vi "电机定位1.1.vi"(0 "VISA I":refnum<visa-resource-name>, 1 "等待时间(ms)":u32=40, 2 "细分设置":dbl=8.0, 3 "电机急停":bool, 4 "X":dbl, 5 "精度":dbl=0.001, 6 "pulDDR2Length":u32, 8 "hDevice":i32, 10 "M-length":dbl, 12 "N-length":dbl) -> (13 "hDevice out":i32, 14 "VISA O":refnum<visa-resource-name>, 18 "X":dbl, 19 "Y":dbl)   [LabVIEW 2016]
uses:
  <vilib>/Analysis/2dsp.llb/Real FFT.vi
  <vilib>/Analysis/4window.llb/Gaussian Window (DBL).vi
  <vilib>/Utility/file.llb/Write Delimited Spreadsheet (DBL).vi
  <vilib>/Utility/file.llb/Read Delimited Spreadsheet (DBL).vi
  <vilib>/Analysis/NI_AALBase.lvlib
  <vilib>/Analysis/NI_AALPro.lvlib
panel:
  out "有效值":dbl
  out "空扫底噪":cdb[](array[numeric])
  out "采集卡底噪":cdb[](array[numeric])
  in  "保存信号":bool
  out "幅频谱":dbl[](graph)
  out "时域谱":dbl[](graph)
  in  "查询信号":bool
  in  "Y":dbl
  in  "确定":bool
  in  "ESC":bool
  # "时域谱"
  # "频域谱"
  # "目标位置"
  # "实时位置"
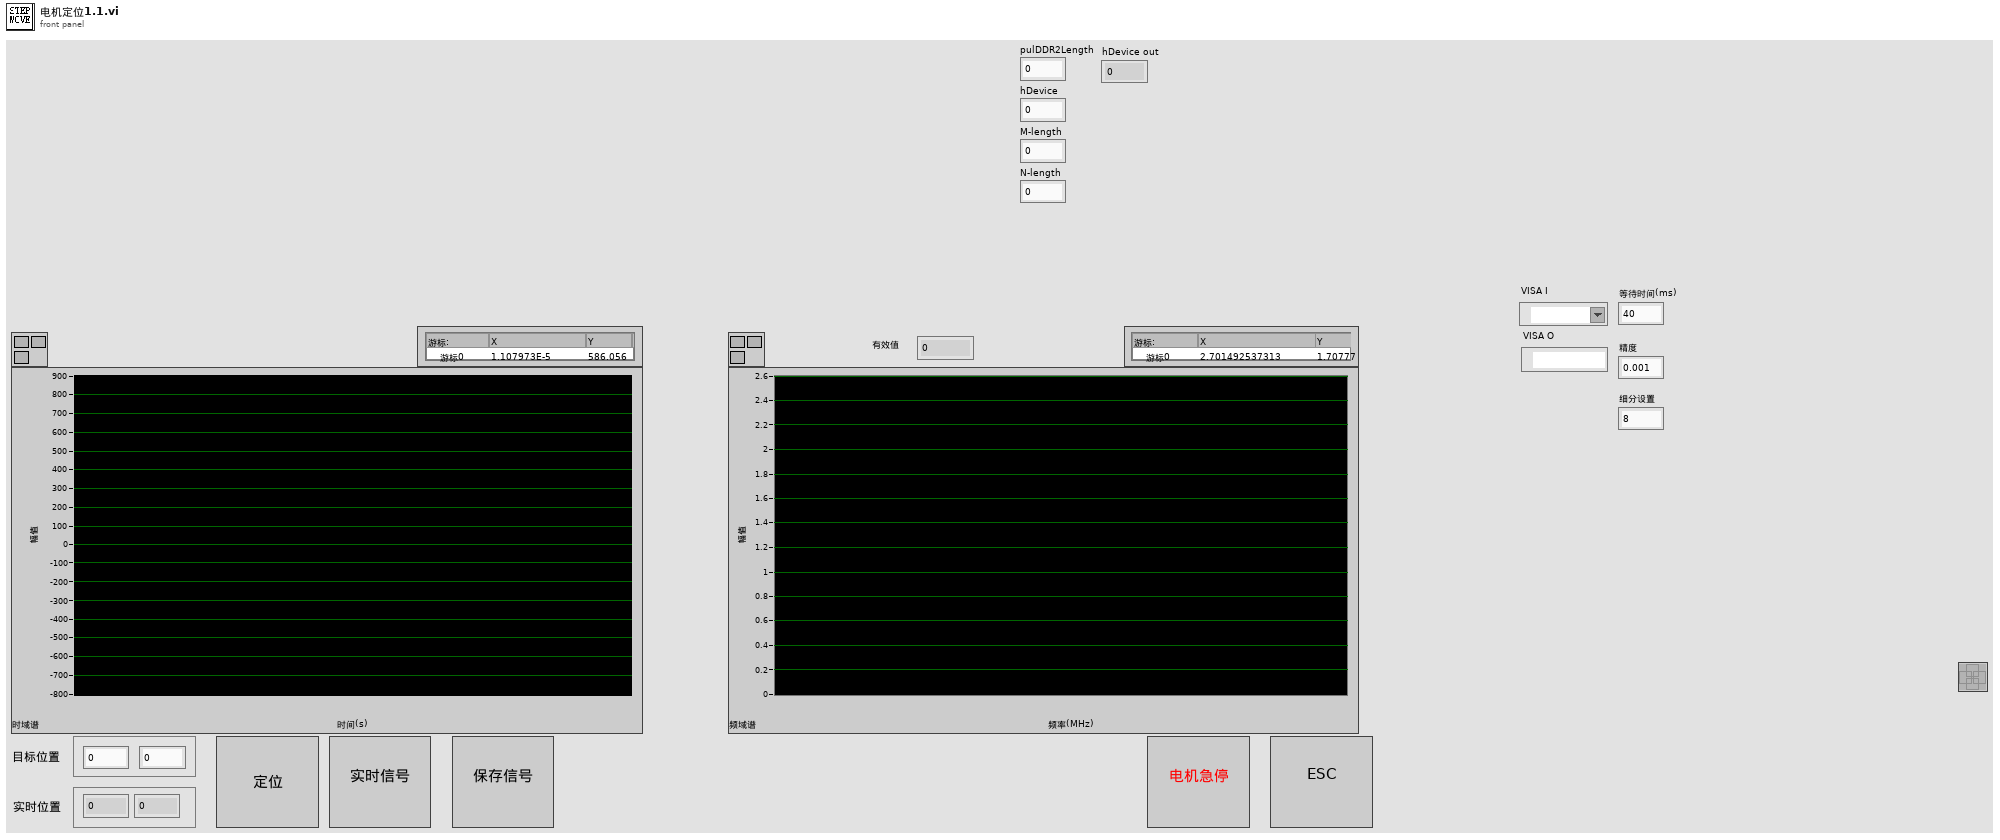
[diagram p1: front panel]
types:
  T1 = enum16{"open", "replace", "create", "open or create", "replace or create", "replace or create with confirmation"}
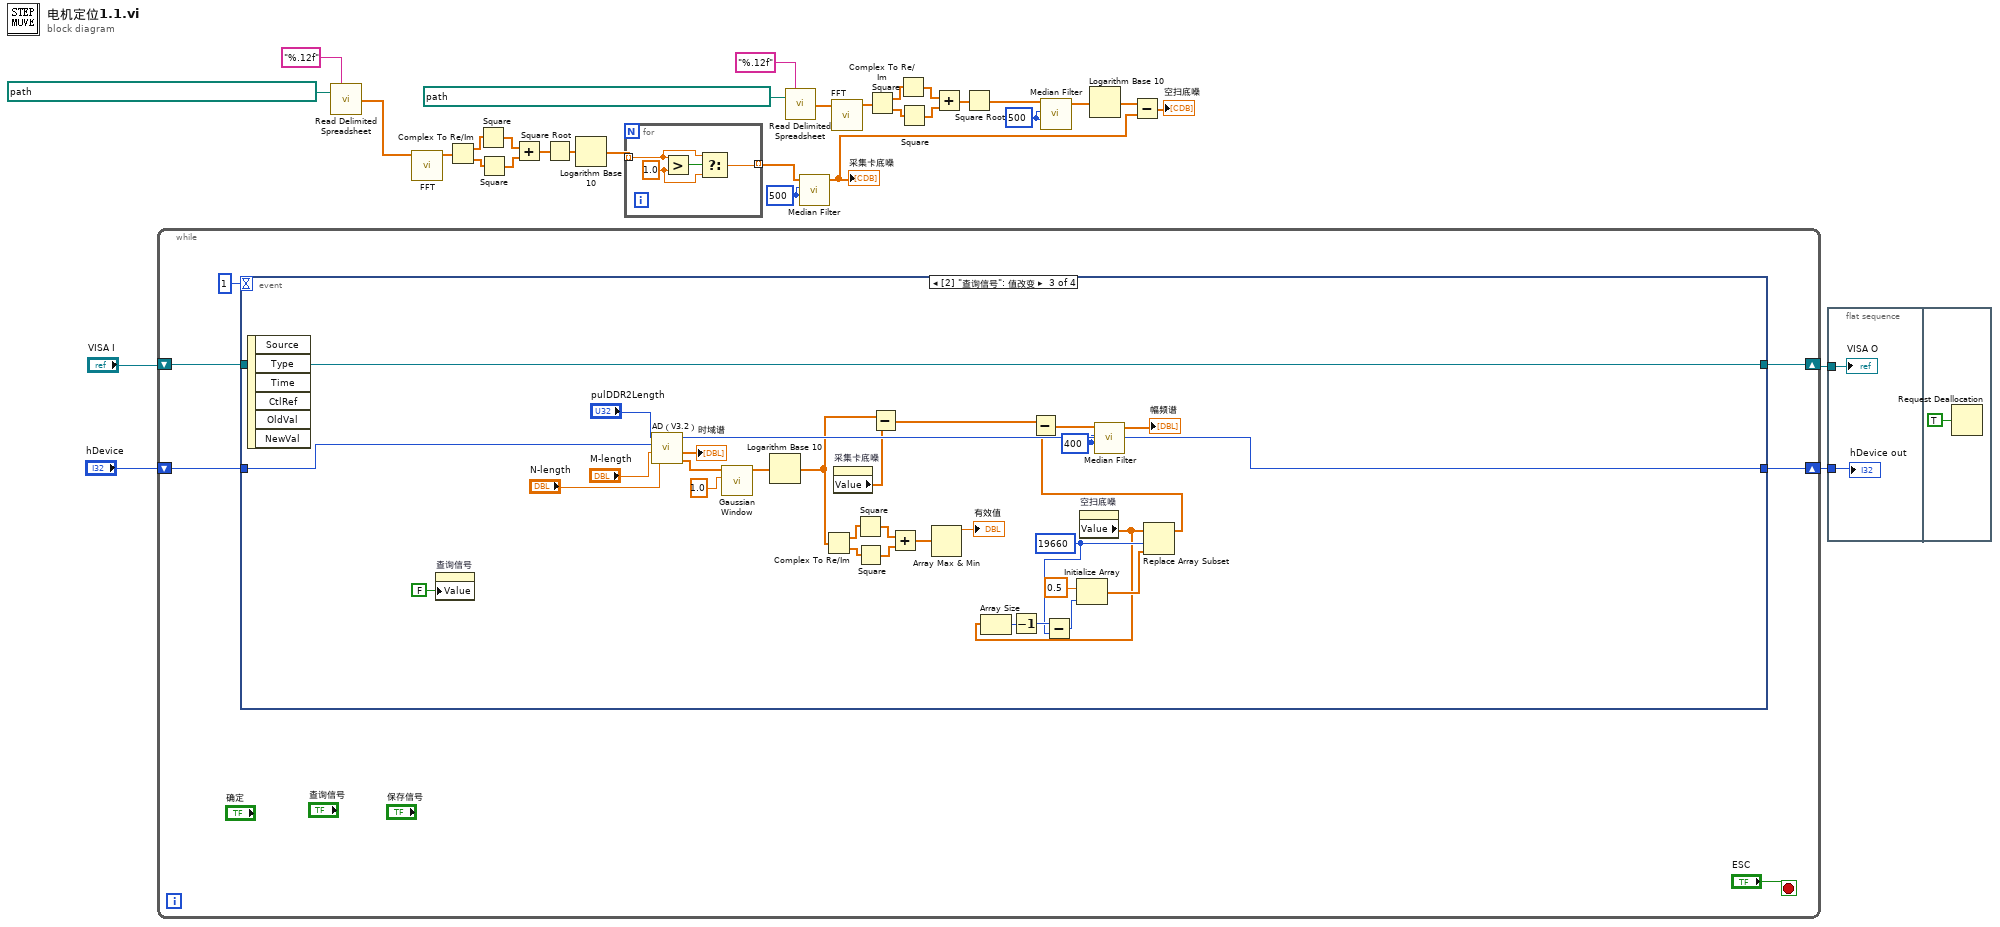
[diagram p0: block diagram]
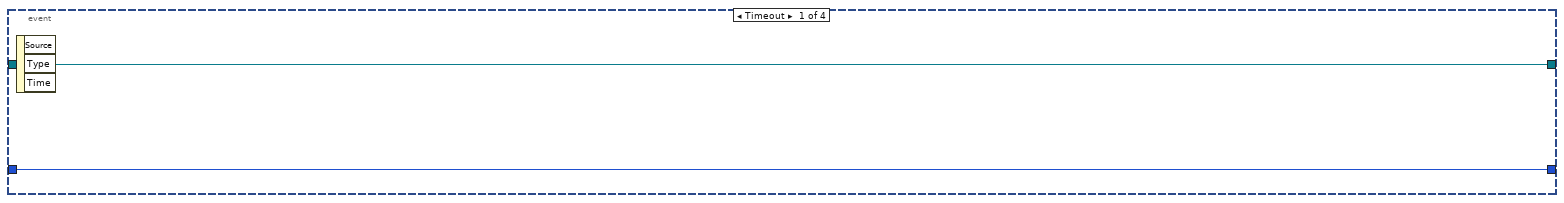
[diagram p2: hidden frame]
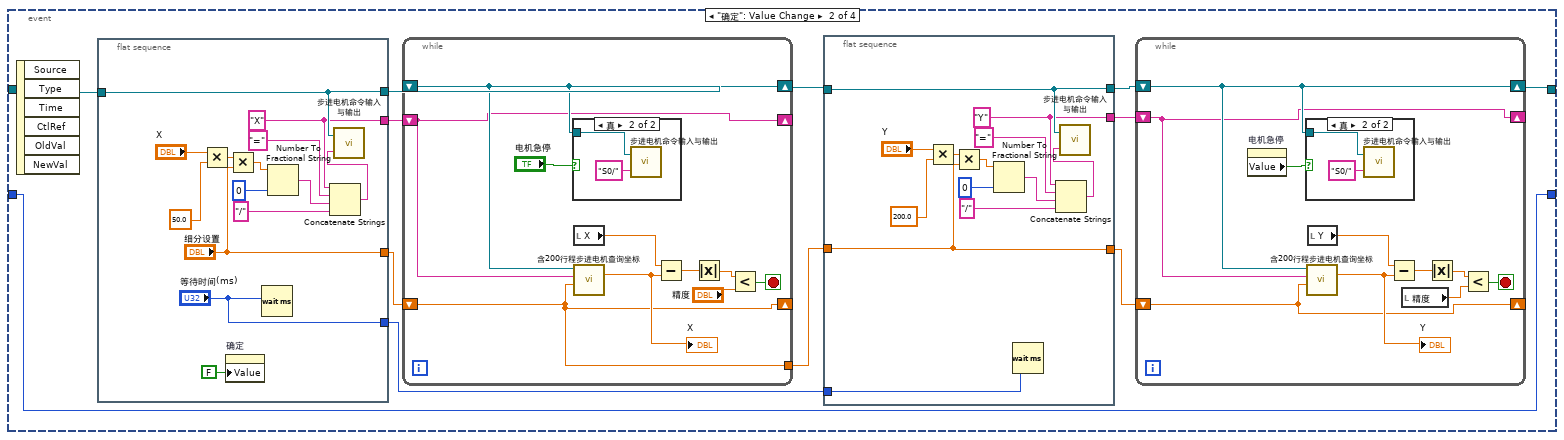
[diagram p3: hidden frame]
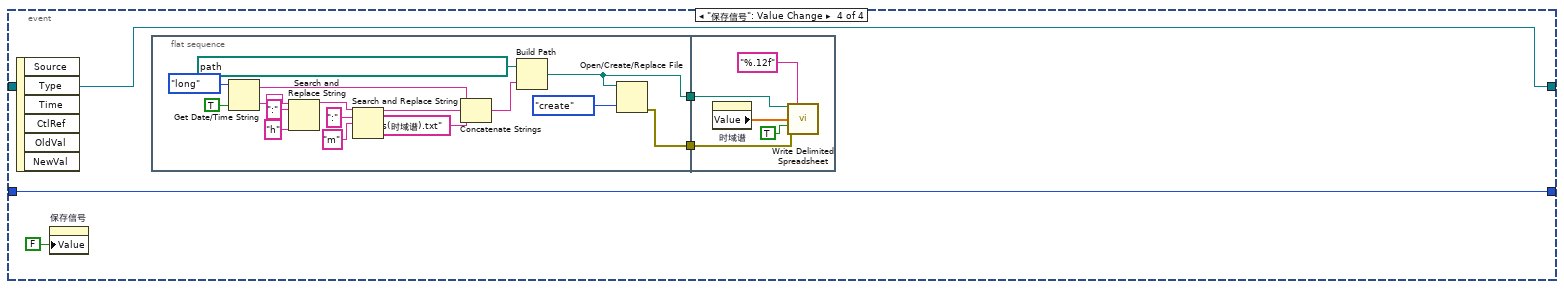
[diagram p6: hidden frame]
diagram:
  w8 = 500 ("left rank")
  w26 = 500 ("left rank")
  n1 = while {
    shift-right: [w37] -> w32
    shift-left: "VISA I" -> [w38]
    shift-right: [w34] -> w29
    shift-left: "hDevice" -> [w35]
    stop <- "ESC" stop-if-true
    n2 = event shown="[2] \"查询信号\": 值改变" {
      selector: _ -> [_ _ _ _]
      dyn-events: _ -> [_ _ _ _]
      timeout: 1 -> [_ _ _ _]
      tunnel: w38 -> [w40 w52 w134 w138]
      tunnel: [w40 w51 w134 w138] -> w37
      tunnel: w35 -> [w39 w41 w130 w137]
      tunnel: [w39 w41 w129 w137] -> w34
      event Timeout {
        n3 = event-data() -> ()  [unwired: 1 in, 3 out]
      }
      event "确定": Value Change {
        n4 = event-data() -> ()  [unwired: 1 in, 6 out]
        n5 = flat-sequence {
          tunnel: w52 -> [w95]
          tunnel: [w95] -> w50
          tunnel: ["细分设置"] -> w49
          tunnel: [w92] -> w48
          tunnel: ["等待时间(ms)"] -> w43
          frame #0 {
            w92 = "X"
            n6 = Multiply(x="X", y=50.0 ("x")) -> (x*y=w98:dbl)
            n7 = property on="确定" class="Bool (严格)"("Value"=FALSE ("确定")) -> ()  [unwired: 2 in, 2 out]
            n8 = Multiply(x=w98, y="细分设置") -> (x*y=w103:dbl)
            n9 = Wait (ms)(milliseconds to wait="等待时间(ms)") -> ()  [unwired: 1 out]
            n10 = Number To Fractional String(number=w103, precision (6)=i16 0 ("精度(6)")) -> (F-format string=w101:string)  [unwired: 2 out]
            n11 = Concatenate Strings(w92, "=" ("字符串"), w101, "/" ("字符串")) -> (w97:string)
            n12 = call "步进电机命令输入与输出.vi"("输入字符串"=w97, "串口通信端口"=w95) -> ()  [unwired: 1 out]
          }
        }
        n13 = while {
          tunnel: [w78] -> w42
          shift-right: [w84] -> w44
          shift-left: w50 -> [w84]
          shift-right: [w79] -> _
          shift-left: w48 -> [w79]
          shift-right: [w78] -> _
          shift-left: w49 -> [w78]
          stop <- w87 stop-if-true
          n14 = case shown="真" "电机急停" {
            tunnel: w84 -> [_ w88]
            frame False {
            }
            frame True {
              n15 = call "步进电机命令输入与输出.vi"("输入字符串"="S0/", "串口通信端口"=w88) -> ()  [unwired: 1 out]
            }
          }
          n16 = local read "X"() -> (w82:dbl)
          n17 = call "含200行程步进电机查询坐标.vi"("细分设置"=w78, "查询坐标轴"=w79, "串口通信端口"=w84) -> ("坐标(mm)"=w81:dbl)  [unwired: 8 in]
          "X" <- w81
          n18 = Subtract(x=w82, y=w81) -> (x-y=w86:dbl)
          n19 = Absolute Value(x=w86) -> (abs(x)=w85:dbl)
          n20 = Less?(x=w85, y="精度") -> (x < y?=w87:bool)
        }
        n21 = flat-sequence {
          tunnel: w44 -> [w69]
          tunnel: [w69] -> w47
          tunnel: [w65] -> w46
          tunnel: [w67] -> w45
          tunnel: w43 -> [w66]
          tunnel: w42 -> [w65]
          frame #0 {
            w67 = "Y"
            n22 = Multiply(x="Y", y=200.0 ("x")) -> (x*y=w72:dbl)
            n23 = Multiply(x=w72, y=w65) -> (x*y=w77:dbl)
            n24 = Number To Fractional String(number=w77, precision (6)=i16 0 ("精度(6)")) -> (F-format string=w75:string)  [unwired: 2 out]
            n25 = Wait (ms)(milliseconds to wait=w66) -> ()  [unwired: 1 out]
            n26 = Concatenate Strings(w67, "=" ("字符串"), w75, "/" ("字符串")) -> (w71:string)
            n27 = call "步进电机命令输入与输出.vi"("输入字符串"=w71, "串口通信端口"=w69) -> ()  [unwired: 1 out]
          }
        }
        n28 = while {
          shift-right: [w59] -> w51
          shift-left: w47 -> [w59]
          shift-right: [w54] -> _
          shift-left: w45 -> [w54]
          shift-right: [w53] -> _
          shift-left: w46 -> [w53]
          stop <- w62 stop-if-true
          n29 = property on="电机急停" class="Bool (严格)"() -> ("Value"=w55:bool)  [unwired: 2 in, 2 out]
          n30 = case shown="真" w55 {
            tunnel: w59 -> [_ w63]
            frame False {
            }
            frame True {
              n31 = call "步进电机命令输入与输出.vi"("输入字符串"="S0/", "串口通信端口"=w63) -> ()  [unwired: 1 out]
            }
          }
          n32 = call "含200行程步进电机查询坐标.vi"("细分设置"=w53, "查询坐标轴"=w54, "串口通信端口"=w59) -> ("坐标(mm)"=w57:dbl)  [unwired: 8 in]
          "Y" <- w57
          n33 = local read "Y"() -> (w58:dbl)
          n34 = Subtract(x=w58, y=w57) -> (x-y=w61:dbl)
          n35 = local read "精度"() -> (w56:dbl)
          n36 = Absolute Value(x=w61) -> (abs(x)=w60:dbl)
          n37 = Less?(x=w60, y=w56) -> (x < y?=w62:bool)
        }
      }
      event "查询信号": Value Change {
        w109 = 19660 ("索引")
        w127 = 400 ("left rank")
        n38 = event-data() -> ()  [unwired: 1 in, 6 out]
        n39 = property on="查询信号" class="Bool (严格)"("Value"=FALSE ("查询信号")) -> ()  [unwired: 2 in, 2 out]
        n40 = call "AD（V3.2）.vi"("N-length"="N-length", "M-length"="M-length", "hDevice"=w130, "pulDDR2Length"="pulDDR2Length") -> ("幅频谱"=w114:dbl[], "时域谱"=→"时域谱":dbl[], "hDevice out"=w129:i32)  [unwired: 5 in]
        n41 = call-poly <vilib>:"Gaussian Window.vi"("standard deviation"=1.0, "X"=w114) -> ("Windowed X"=w113:dbl[])  [unwired: 8 in, 1 out]
        n42 = Logarithm Base 10(1:w113) -> (0:w117:dbl[])
        n43 = Complex To Re/Im(x + iy=w117) -> (x=w122:dbl[], y=w123:dbl[])
        n44 = property on="采集卡底噪" class="Arr (严格)"() -> ("Value"=w116:cdb[])  [unwired: 2 in, 2 out]
        n45 = Square(x=w122) -> (x^2=w124:dbl[])
        n46 = Square(x=w123) -> (x^2=w125:dbl[])
        n47 = Subtract(x=w117, y=w116) -> (x-y=w119:cdb[])
        n48 = Add(x=w124, y=w125) -> (x+y=w121:dbl[])
        n49 = Array Max & Min(array=w121) -> (max value=→"有效值":dbl)  [unwired: 3 out]
        n50 = property on="空扫底噪" class="Arr (严格)"() -> ("Value"=w106:cdb[])  [unwired: 2 in, 2 out]
        n51 = Array Size(array=w106) -> (size(s)=w111:i32)
        n52 = Decrement(x=w111) -> (x-1=w110:i32)
        n53 = Subtract(x=w110, y=w109) -> (x-y=w108:i32)
        n54 = Initialize Array(0.5 ("元素"), w108) -> (w107:dbl[])
        n55 = Replace Array Subset(array=w106, new element=w107, index=w109) -> (w105:cdb[])
        n56 = Subtract(x=w119, y=w105) -> (x-y=w115:cdb[])
        n57 = call <vilib>:"Median Filter.vi"("right rank"=w127, "left rank"=w127, "X"=w115) -> ("Filtered X"=→"幅频谱":dbl[])  [unwired: 7 in, 1 out]
      }
      event "保存信号": Value Change {
        n58 = event-data() -> ()  [unwired: 1 in, 6 out]
        n59 = property on="保存信号" class="Bool (严格)"("Value"=FALSE ("保存信号")) -> ()  [unwired: 2 in, 2 out]
        n60 = flat-sequence {
          tunnel: [w153] -> w136
          tunnel: [w152] -> w135
          tunnel: w136 -> [w157]
          tunnel: w135 -> [w156]
          frame #0 {
            n61 = Get Date/Time String(date format (0)=enum16{"short", "long", "abbreviated"}."long" ("日期格式(0)"), want seconds? (F)=TRUE ("需要秒？(F)")) -> (date string=w144:string, time string=w145:string)  [unwired: 1 in]
            n62 = Search and Replace String(input string=w145, search string=":" ("搜索字符串"), replace string="h" ("替换字符串(\"\")")) -> (result string=w150:string)  [unwired: 5 in, 3 out]
            n63 = Search and Replace String(input string=w150, search string=":" ("搜索字符串"), replace string="m" ("替换字符串(\"\")")) -> (result string=w143:string)  [unwired: 5 in, 3 out]
            n64 = Concatenate Strings(w144, w143, "s(时域谱).txt" ("字符串")) -> (w142:string)
            n65 = Build Path(base path=path "C:/Users/H301/Desktop/art采集实验数据/单点时域谱" ("基路径"), name or relative path=w142) -> (appended path=w153:path)
            n66 = Open/Create/Replace File(file path (use dialog)=w153, operation (0:open)=T1."create" ("操作(0:open)")) -> (error out=w152:errorcluster)  [unwired: 4 in, 2 out]
          }
          frame #1 {
            n67 = property on="时域谱" class="WFGraph (严格)"() -> ("Value"=w158:dbl[])  [unwired: 2 in, 2 out]
            n68 = call-poly <vilib>:"Write Delimited Spreadsheet.vi"("file path (dialog if empty)"=w157, "format (%.3f)"="%.12f", "1D data"=w158, "append to file? (new file:F)"=TRUE, "error in (no error)"=w156) -> ()  [unwired: 9 in, 2 out]
          }
        }
      }
    }
  }
  n69 = call-poly <vilib>:"Read Delimited Spreadsheet.vi"("file path (dialog if empty)"=path "C:/Users/H301/Desktop/art采集实验数据/采集卡均值底噪.txt", "format (%.3f)"="%.12f") -> ("first row"=w9:dbl[])  [unwired: 8 in, 5 out]
  n70 = call-poly <vilib>:"FFT.vi"("X"=w9) -> ("FFT {X}"=w12:cdb[])  [unwired: 9 in, 1 out]
  n71 = Complex To Re/Im(x + iy=w12) -> (x=w10:dbl[], y=w11:dbl[])
  n72 = Square(x=w10) -> (x^2=w13:dbl[])
  n73 = Square(x=w11) -> (x^2=w14:dbl[])
  n74 = Add(x=w13, y=w14) -> (x+y=w15:dbl[])
  n75 = Square Root(x=w15) -> (sqrt(x)=w6:dbl[])
  n76 = Logarithm Base 10(1:w6) -> (0:w5:dbl[])
  n77 = for {
    tunnel: w5 -> [w162] mode=indexing
    tunnel: [w161] -> w7 mode=indexing
    w163 = 1.0 ("y")
    n78 = Greater?(x=w162, y=w163) -> (0:w164:bool)
    n79 = Select(t=w162, s=w164, f=w163) -> (s? t:f=w161:dbl)
  }
  n80 = call-poly <vilib>:"Read Delimited Spreadsheet.vi"("file path (dialog if empty)"=path "C:/Users/H301/Desktop/art采集实验数据/信号源均值底噪.txt", "format (%.3f)"="%.12f") -> ("first row"=w25:dbl[])  [unwired: 8 in, 5 out]
  n81 = call <vilib>:"Median Filter.vi"("right rank"=w8, "left rank"=w8, "X"=w7) -> ("Filtered X"=w2:dbl[])  [unwired: 7 in, 1 out]
  "采集卡底噪" <- w2
  n82 = call-poly <vilib>:"FFT.vi"("X"=w25) -> ("FFT {X}"=w20:cdb[])  [unwired: 9 in, 1 out]
  n83 = Complex To Re/Im(x + iy=w20) -> (x=w22:dbl[], y=w21:dbl[])
  n84 = Square(x=w22) -> (x^2=w19:dbl[])
  n85 = Square(x=w21) -> (x^2=w18:dbl[])
  n86 = Add(x=w19, y=w18) -> (x+y=w17:dbl[])
  n87 = Square Root(x=w17) -> (sqrt(x)=w16:dbl[])
  n88 = call <vilib>:"Median Filter.vi"("right rank"=w26, "left rank"=w26, "X"=w16) -> ("Filtered X"=w4:dbl[])  [unwired: 7 in, 1 out]
  n89 = Logarithm Base 10(1:w4) -> (0:w3:dbl[])
  n90 = Subtract(x=w3, y=w2) -> (x-y=→"空扫底噪":dbl[])
  n91 = flat-sequence {
    tunnel: w32 -> [w166]
    tunnel: w29 -> [w165]
    frame #0 {
      "VISA O" <- w166
      "hDevice out" <- w165
    }
    frame #1 {
      n92 = Request Deallocation(TRUE ("标志")) -> ()
    }
  }
